vi "Primitives.vi"(1 "Angle to Target":i32, 2 "Bump 1":bool, 3 "Bump 2":bool, 5 "Primitive":string, 8 "Distance to Target":i32) -> (0 "Port Speed":i32, 6 "Starboard Speed":i32)   [LabVIEW 2012]
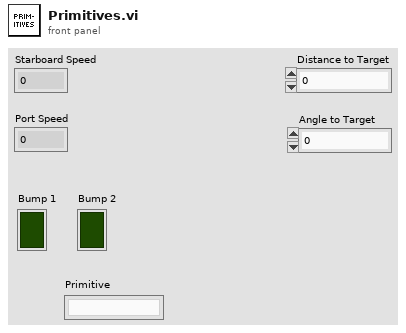
[diagram p1: front panel]
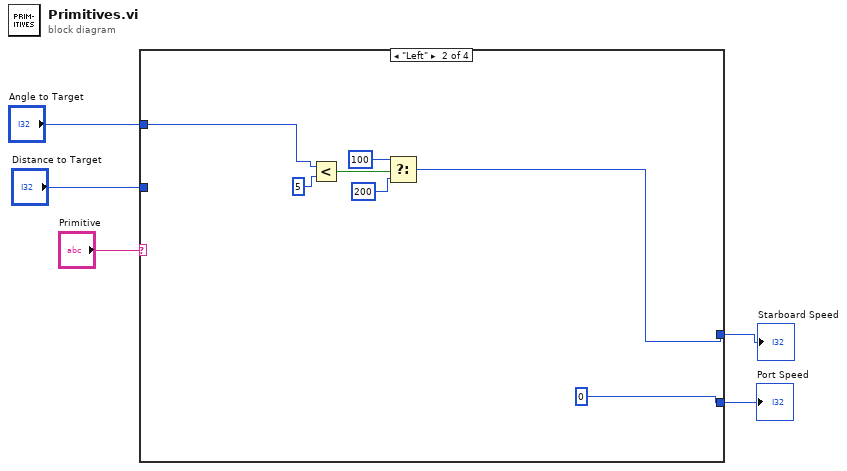
[diagram p0: block diagram]
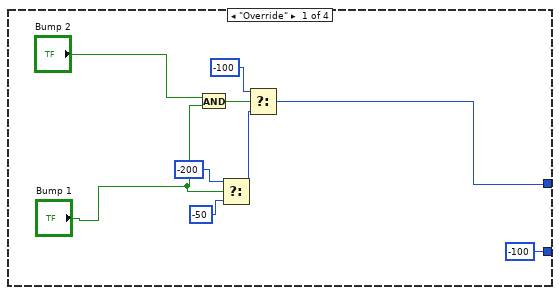
[diagram p2: hidden frame]
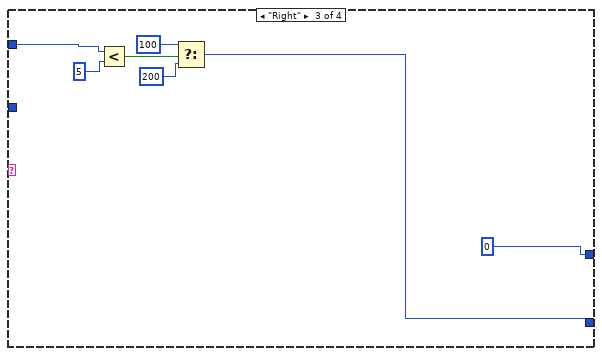
[diagram p3: hidden frame]
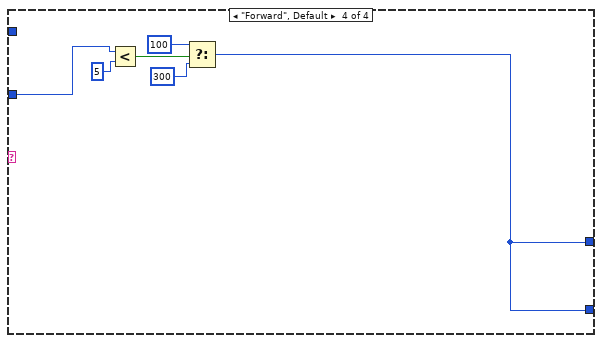
[diagram p4: hidden frame]
diagram:
  n1 = case shown="\"Left\"" "Primitive" {
    tunnel: [w12 w15 0 w31] -> w4
    tunnel: [-100 0 w22 w31] -> w3
    tunnel: "Angle to Target" -> [_ w16 w23 _]
    tunnel: "Distance to Target" -> [_ _ _ w34]
    frame "Override" {
      n2 = And(x="Bump 2", y="Bump 1") -> (x .and. y?=w14:bool)
      n3 = Select(t=-200, s="Bump 1", f=-50) -> (s? t:f=w11:i32)
      n4 = Select(t=-100, s=w14, f=w11) -> (s? t:f=w12:i32)
    }
    frame "Left" {
      n5 = Less?(x=w16, y=5) -> (x < y?=w19:bool)
      n6 = Select(t=100, s=w19, f=200) -> (s? t:f=w15:i32)
    }
    frame "Right" {
      n7 = Less?(x=w23, y=5) -> (x < y?=w26:bool)
      n8 = Select(t=100, s=w26, f=200) -> (s? t:f=w22:i32)
    }
    frame "Forward", Default {
      n9 = Less?(x=w34, y=5) -> (x < y?=w32:bool)
      n10 = Select(t=100, s=w32, f=300) -> (s? t:f=w31:i32)
    }
  }
  "Starboard Speed" <- w4
  "Port Speed" <- w3
